vi "ExSimple.vi"() -> ()   [LabVIEW 2016]
uses:
  <vilib>/Math Plots/3D Math Plots/3D Surface/3D Surface XCtrl/3D Surface.xctl
  <vilib>/Math Plots/3D Math Plots/3D Surface/3D Surface Datatype/Public/Plot Helper (Vector).vi
  <vilib>/Math Plots/3D Math Plots/3D Surface/3D Surface Datatype/3D Surface Datatype.lvclass
panel:
  in  "Save flle":path
  in  "Save":bool
  in  "nm/pixel":dbl=0.101
  in  "Start wavelength":dbl=606.0
  out "XY Graph":cluster{"Array - Numeric":dbl[], dbl[]}[](graph)
  out "max value":dbl format="%#_6p"
  out "3D Surface":refnum<class "3D Plot Datatype.lvclass">[](xcontrol)
  out "Temperature 2":dbl caption="Temperature out"
  out "Intensity Graph":u16[][](graph)
  in  "Exposure":dbl=0.001 format="%.3f"
  in  "Close Compensation time ms 2":u32=8
  in  "Open Compensation time ms":u32=8
  in  "Temperature":dbl format="%.2f"
  out "error out":errorcluster
  in  "error in (no error)":errorcluster
  # "Note: for the Cascade and\nPhotonMax the open/close\n compensation should be 0"
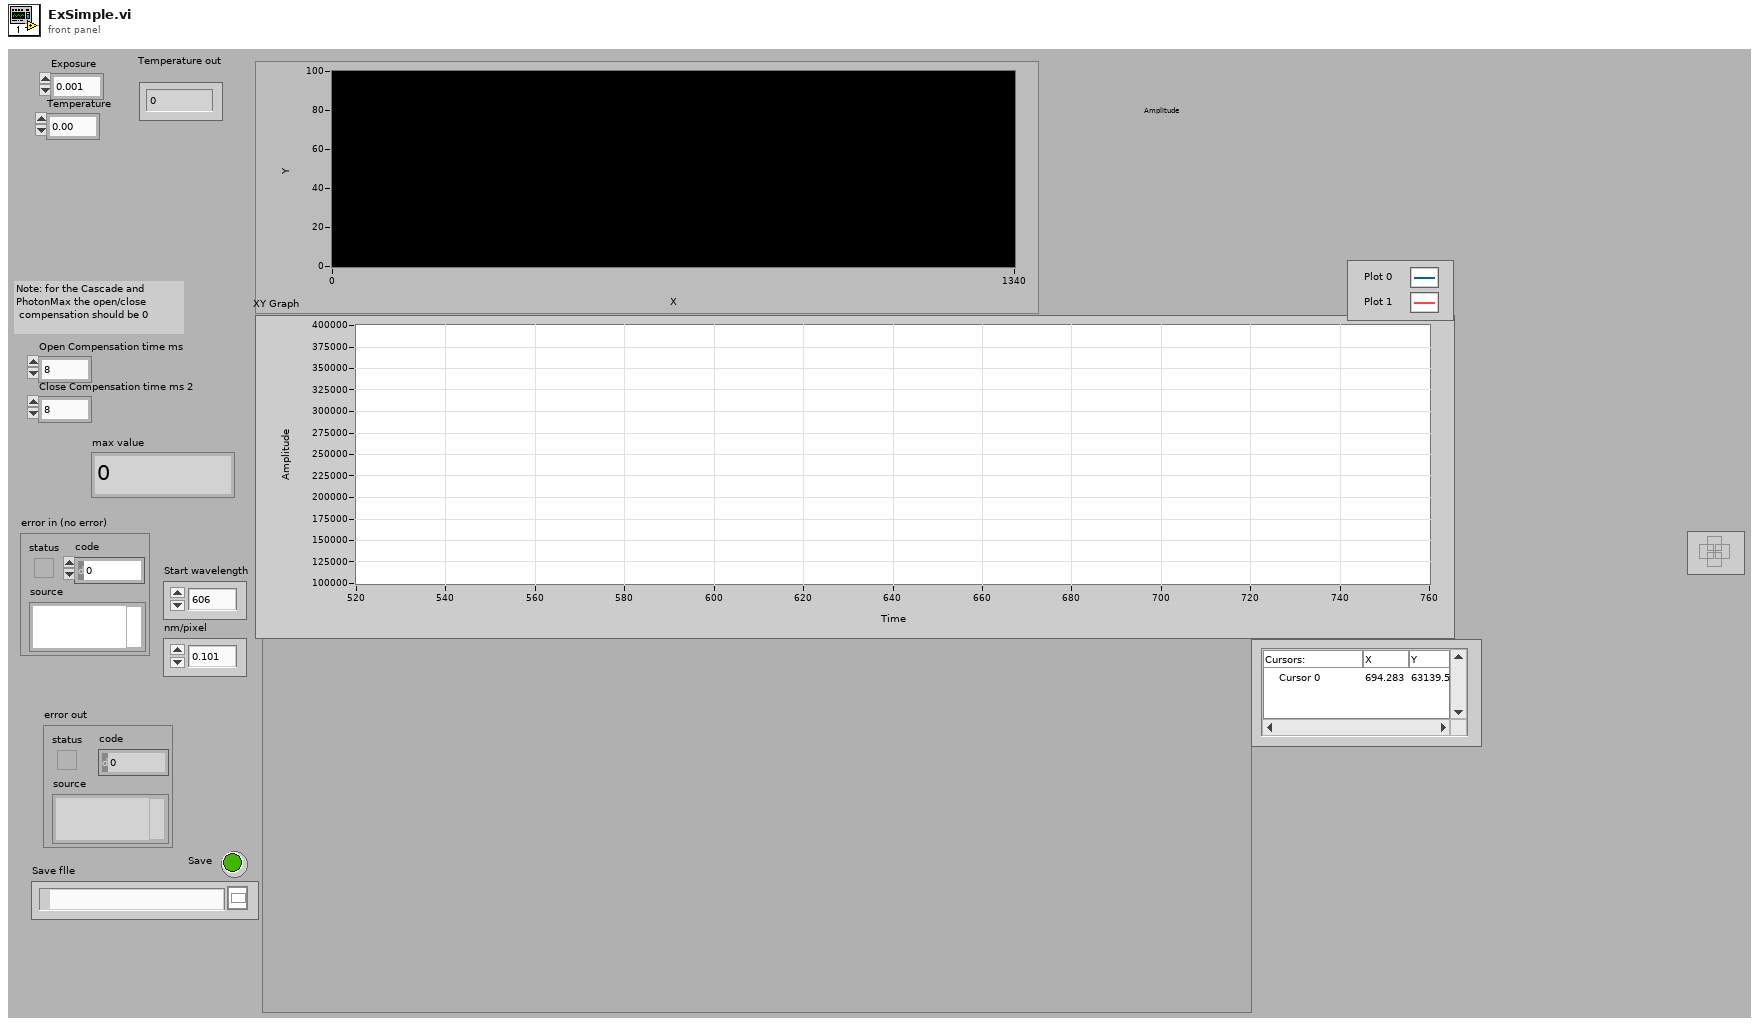
[diagram p1: front panel]
types:
  T1 = cluster{"Open Compensation time ms":u32, "Close Compensation time ms 2":u32}
  T2 = cluster{"Camera Handle":u32, "File Handle":u32, "Image Handle":u32}
  T3 = enum16{"open", "open or create", "create or replace", "create", "open (read-only)"}
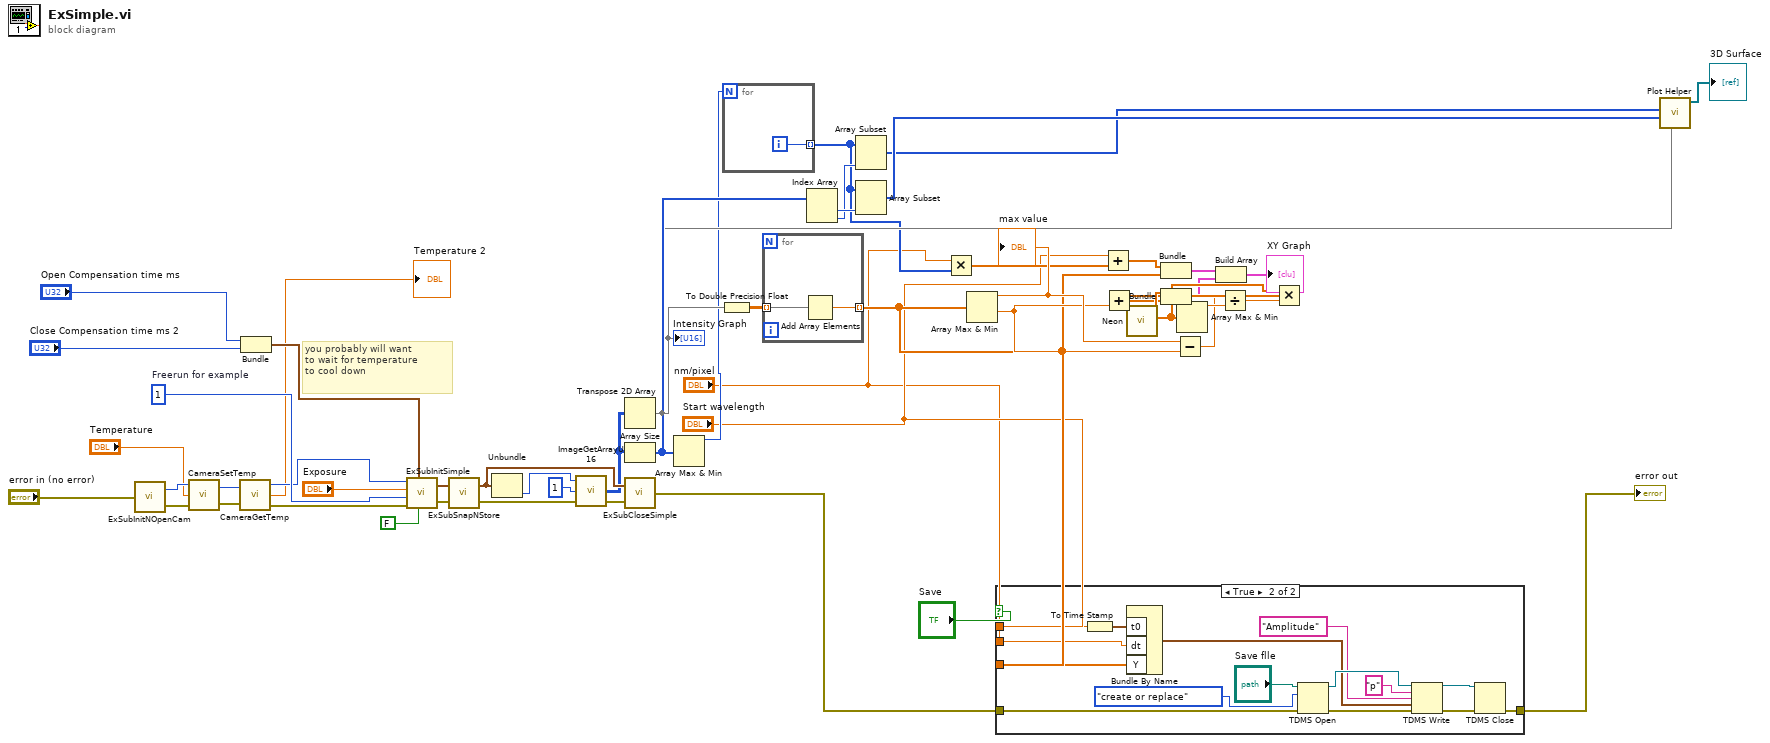
[diagram p0: block diagram]
diagram:
  w42 = 1  # Freerun for example
  # "you probably will want \nto wait for temperature \nto cool down"
  n1 = call "ExSubInitNOpenCam.vi"("error in (no error)"="error in (no error)") -> ("Camera Handle"=w51:u32, "error out"=w52:errorcluster)
  n2 = call <userlib>:"CameraSetTemp.vi"("error in (no error)"=w52, "Temperature"="Temperature", "Camera Handle"=w51) -> ("error out"=w36:errorcluster, "Camera Handle"=w33:u32)
  n3 = call <userlib>:"CameraGetTemp.vi"("Camera Handle"=w33, "error in (no error)"=w36) -> ("Camera Handle"=w34:u32, "Temperature"=→"Temperature 2":dbl, "error out"=w35:errorcluster)
  n4 = Bundle("Open Compensation time ms"="Open Compensation time ms", "Close Compensation time ms 2"="Close Compensation time ms 2") -> (w45:T1)  [unwired: 1 in]
  n5 = call "ExSubInitSimple.vi"("Intensifier"=FALSE, "Shutter Comp"=w45, "error in (no error)"=w35, "Triggering mode"=w42, "Exposure"="Exposure", "Camera Handle"=w34) -> ("error out"=w48:errorcluster, "Handles"=w49:cluster{"Camera":u32, "File":u32, "Image":u32})
  n6 = call "ExSubSnapNStore.vi"("error in (no error)"=w48, "Handle Cluster"=w49) -> ("error out"=w39:errorcluster, "Handle Cluster Out"=w41:T2)
  n7 = Unbundle(w41) -> ("Image Handle"=w40:u32)  [unwired: 2 out]
  n8 = call <userlib>:"ImageGetArrayU16.vi"("error in"=w39, "Z position"=1, "Image Handle"=w40) -> ("error out"=w38:errorcluster, "Array uint 16"=w30:u16[][])  [unwired: 1 out]
  n9 = Transpose 2D Array(2D array=w30) -> (transposed array=w24:u16[][])
  "Intensity Graph" <- w24
  n10 = Array Size(array=w30) -> (size(s)=w29:i32[])
  n11 = call "ExSubCloseSimple.vi"("error in (no error)"=w38, "Handles In"=w41) -> ("error out"=w4:errorcluster)
  n12 = Array Max & Min(array=w29) -> (max value=w22:i32)  [unwired: 3 out]
  n13 = To Double Precision Float(number=w24) -> (double precision float=w23:dbl[][])
  n14 = for {
    N: w22 -> [_]
    tunnel: [w54] -> w21 mode=indexing
    i -> [w54]
  }
  n15 = for {
    tunnel: w23 -> [w56] mode=indexing
    tunnel: [w55] -> w5 mode=indexing
    n16 = Add Array Elements(numeric array=w56) -> (sum=w55:dbl)
  }
  n17 = Index Array(array=w29) -> (element #1=w28:i32, element #2=w27:i32)  [unwired: 2 in]
  n18 = Array Subset(array=w21, length=w27) -> (w25:i32[])  [unwired: 1 in]
  n19 = Array Subset(array=w21, length=w28) -> (w26:i32[])  [unwired: 1 in]
  n20 = Multiply(x="nm/pixel", y=w21) -> (x*y=w10:dbl[])
  n21 = Array Max & Min(array=w5) -> (max value=w14:dbl, min value=w11:dbl)  [unwired: 2 out]
  "max value" <- w14
  n22 = case shown="True" "Save" {
    tunnel: w5 -> [_ w63]
    tunnel: w4 -> [w57 w70]
    tunnel: [w57 w67] -> w3
    tunnel: "Start wavelength" -> [_ w62]
    tunnel: "nm/pixel" -> [_ w60]
    frame False {
    }
    frame True {
      n23 = To Time Stamp(1:w62) -> (0:w61:timestamp)
      n24 = Bundle By Name("t0"=w61, "dt"=w60, "Y"=w63) -> (w59:waveform(dbl))  [unwired: 1 in]
      n25 = TDMS Open(8:w70, 10:T3."create or replace" ("operation (0:open)"), 11:"Save flle") -> (0:w69:errorcluster, 3:w66:refnum<k34>)  [unwired: 4 in]
      n26 = TDMS Write(0:w66, 5:"p" ("group name in (Untitled)"), 7:"Amplitude" ("channel name(s) in (Untitled)"), 9:w59, 11:w69) -> (4:w65:refnum<k34>, 15:w68:errorcluster)  [unwired: 1 in, 2 out]
      n27 = TDMS Close(8:w68, 11:w65) -> (0:w67:errorcluster)  [unwired: 1 out]
    }
  }
  "error out" <- w3
  n28 = Add(x="Start wavelength", y=w10) -> (x+y=w9:dbl[])
  n29 = call "Neon.vi"() -> ("Array - Numeric 2"=w17:dbl[], "Array - Numeric"=w20:dbl[])  [unwired: 10 in]
  n30 = Bundle(w9, w5) -> (w8:cluster{dbl[], dbl[]})  [unwired: 1 in]
  n31 = Subtract(x=w14, y=w11) -> (x-y=w13:dbl)
  n32 = Array Max & Min(array=w17) -> (max value=w19:dbl)  [unwired: 3 out]
  n33 = Divide(x=w13, y=w19) -> (x/y=w18:dbl)
  n34 = Multiply(x=w17, y=w18) -> (x*y=w16:dbl[])
  n35 = Add(x=w16, y=w11) -> (x+y=w12:dbl[])
  n36 = Bundle("Array - Numeric"=w20, w12) -> (w15:cluster{"Array - Numeric":dbl[], dbl[]})  [unwired: 1 in]
  n37 = Build Array(w8, w15) -> (→"XY Graph":cluster{"Array - Numeric":dbl[], dbl[]}[])
  n38 = call-poly <vilib>:"Plot Helper.vi"("z matrix"=w24, "y vector"=w26, "x vector"=w25) -> ("3D Plot lvclass Array out"=→"3D Surface":refnum<class "3D Plot Datatype.lvclass">[])  [unwired: 3 in, 5 out]
